vi "Create RTU Over TCP Master.vi"(7 "unit ID":u8=1, 8 "error in":errorcluster, 9 "connect timeout ms":i32, 10 "port (502)":u16=502, 11 "address":string) -> (0 "error out":errorcluster, 3 "TCP master instance":refnum<class "Modbus Master.lvclass">)   [LabVIEW 2015]
doc: "Creates a standard TCP master using an RTU transmissiaon data unit. This instance looks for a slave at the <B>address</B> and <B>port</B> specified."
uses:
  <vilib>/NI/Modbus Library/API/Master/Modbus Master.lvclass
  <vilib>/NI/Modbus Library/Network Protocol/Network Master/TCP/TCP Master.lvclass
  <vilib>/NI/Modbus Library/Master Function Definition/Master Function Definition.lvclass
  <vilib>/NI/Modbus Library/Transmission Data Unit/RTU/RTU Data Unit.lvclass
  <vilib>/NI/Modbus Library/Transmission Data Unit/RTU/RTU Data Unit.lvclass/RTU Data Unit.ctl
  <vilib>/NI/Modbus Library/Network Protocol/Network Master/TCP/TCP Master.lvclass/TCP Master.ctl
  <vilib>/NI/Modbus Library/API/Master/Modbus Master.lvclass/Modbus Master.ctl
  <vilib>/NI/Modbus Library/Transmission Data Unit/Transmission Data Unit.lvclass/Transmission Data Unit.ctl
  <vilib>/NI/Modbus Library/API/Modbus API.lvclass/Modbus API.ctl
  <vilib>/NI/Modbus Library/Network Protocol/Network Master/TCP/Write Address.vi
  <vilib>/NI/Modbus Library/Network Protocol/Network Master/TCP/Write Port.vi
  <vilib>/NI/Modbus Library/Network Protocol/Network Master/TCP/Write connect timeout ms.vi
  <vilib>/NI/Modbus Library/API/Modbus API.lvclass
  <vilib>/NI/Modbus Library/Transmission Data Unit/Transmission Data Unit.lvclass
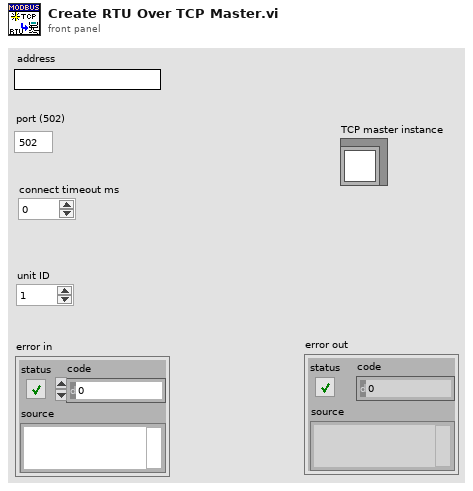
[diagram p1: front panel]
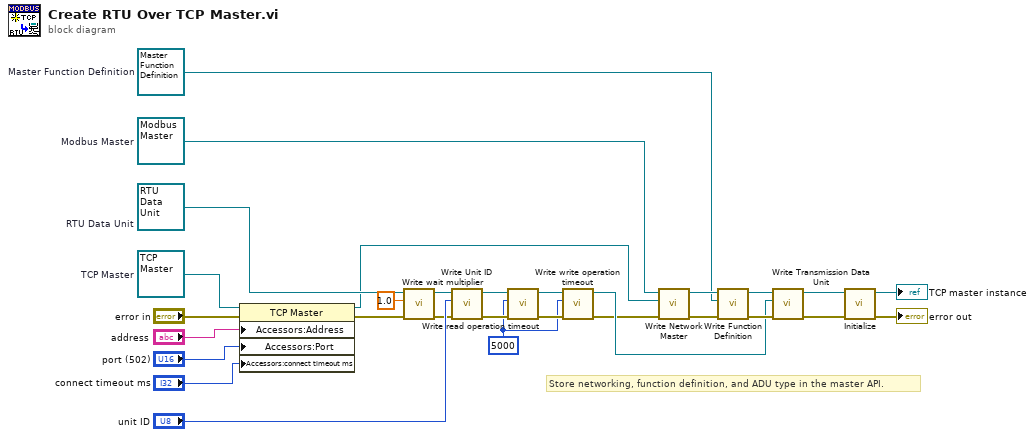
[diagram p0: block diagram]
diagram:
  w1 = 5000 ("read operation timeout")
  w7 = refnum<class "RTU Data Unit.lvclass"> refnum  # RTU Data Unit
  w16 = refnum<class "Master Function Definition.lvclass"> refnum  # Master Function Definition
  w23 = refnum<class "Modbus Master.lvclass"> refnum  # Modbus Master
  w29 = refnum<class "TCP Master.lvclass"> refnum  # TCP Master
  # "Store networking, function definition, and ADU type in the master API."
  n1 = property class="TCP Master"(reference=w29, error in="error in", "Accessors:Address"="address", "Accessors:Port"="port (502)", "Accessors:connect timeout ms"="connect timeout ms") -> (reference out=w3:refnum<class "TCP Master.lvclass">, error out=w4:errorcluster)
  n2 = call <vilib>:"Write wait multiplier.vi"("error in (no error)"=w4, "wait multiplier"=sgl 1.0, "RTU Data Unit in"=w7) -> ("error out"=w8:errorcluster, "RTU Data Unit out"=w15:refnum<class "RTU Data Unit.lvclass">)  [unwired: 7 in]
  n3 = call <vilib>:"Write Unit ID.vi"("error in"=w8, "unit ID"="unit ID", "transmission data unit in"=w15) -> ("error out"=w11:errorcluster, "transmission data unit out"=w12:refnum<class "RTU Data Unit.lvclass">)  [unwired: 7 in]
  n4 = call <vilib>:"Write read operation timeout.vi"("error in (no error)"=w11, "read operation timeout"=w1, "transmission data unit in"=w12) -> ("error out"=w10:errorcluster, "transmission data unit out"=w13:refnum<class "RTU Data Unit.lvclass">)  [unwired: 7 in]
  n5 = call <vilib>:"Write write operation timeout.vi"("error in (no error)"=w10, "write operation timeout"=w1, "transmission data unit in"=w13) -> ("error out"=w2:errorcluster, "transmission data unit out"=w9:refnum<class "RTU Data Unit.lvclass">)  [unwired: 7 in]
  n6 = call <vilib>:"Write Network Master.vi"("error in"=w2, "network master"=w3, "Modbus master in"=w23) -> ("error out"=w17:errorcluster, "Modbus master out"=w22:refnum<class "Modbus Master.lvclass">)  [unwired: 7 in]
  n7 = call <vilib>:"Write Function Definition.vi"("error in"=w17, "master function definition"=w16, "Modbus master in"=w22) -> ("error out"=w18:errorcluster, "Modbus master out"=w21:refnum<class "Modbus Master.lvclass">)  [unwired: 7 in]
  n8 = call <vilib>:"Write Transmission Data Unit.vi"("error in"=w18, "transmission data unit"=w9, "Modbus instance in"=w21) -> ("error out"=w19:errorcluster, "Modbus instance out"=w20:refnum<class "Modbus Master.lvclass">)  [unwired: 7 in]
  n9 = call-dynamic "Initialize.vi"("error in"=w19, "Modbus master in"=w20) -> ("error out"=→"error out":errorcluster, "Modbus master out"=→"TCP master instance":refnum<class "Modbus Master.lvclass">)  [unwired: 8 in]
